vi "Screen Caps VI.vi"() -> ()   [LabVIEW 2015]
uses:
  Circle cluster.ctl
  colors.ctl
  Circle/Circle.lvclass
  Shape/Shape.lvclass/Shape.ctl
  Circle Library.lvlib
  Shape/Shape.lvclass
panel:
  out "area":dbl
  out "area":dbl
  in  "error in (no error)":errorcluster
  out "output cluster":T1
  in  "Radius":dbl
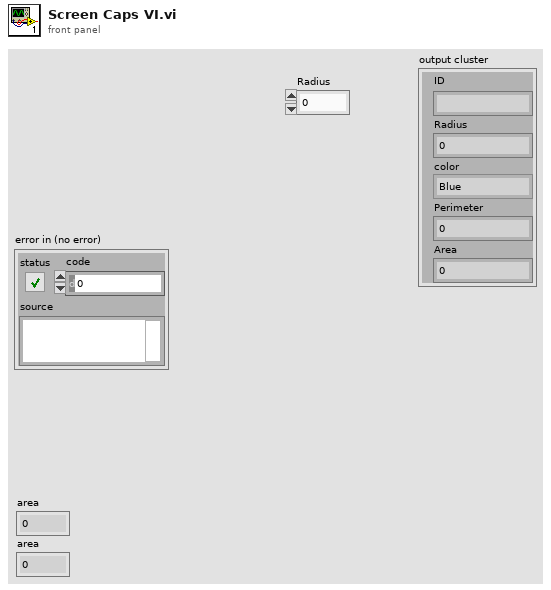
[diagram p1: front panel]
types:
  T1 = typedef "Circle Library.lvlib/Circle cluster.ctl" = cluster{"ID":string, "Radius":dbl, "color":T2, "Perimeter":dbl, "Area":dbl}
  T2 = typedef "colors.ctl" = enum16{"Blue", "Red", "Green", "Yellow"}
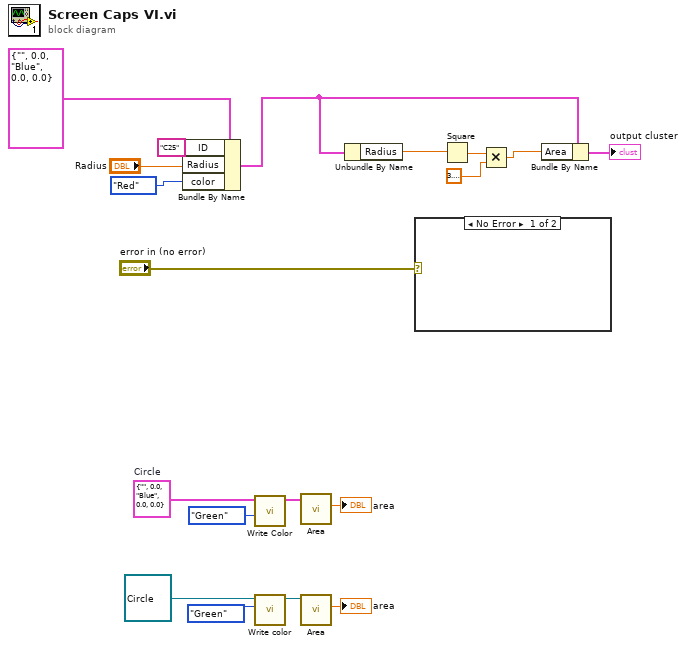
[diagram p0: block diagram]
diagram:
  w6 = T1 {"ID"="", "Radius"=0.0, "color"=enum."Blue", "Perimeter"=0.0, "Area"=0.0}  # Circle
  n1 = Bundle By Name(cluster=T1 {"ID"="", "Radius"=0.0, "color"=enum."Blue", "Perimeter"=0.0, "Area"=0.0} ("Circle"), "ID"="C25", "Radius"="Radius", "color"=colors."Red") -> (w13:T1)
  n2 = call "Write Color.vi"("color"=colors."Green", "Circle"=w6) -> ("Circle 2"=w5:T1)  [unwired: 9 in]
  n3 = call "Write color.vi"("color"=colors."Green", "Shape in"=refnum<class "Circle.lvclass"> refnum ("Circle.lvclass")) -> ("Shape out"=w2:refnum<class "Circle.lvclass">)  [unwired: 8 in, 1 out]
  n4 = call "Area.vi"("Circle in"=w5) -> ("Area"=→"area":dbl)  [unwired: 9 in, 1 out]
  n5 = call-dynamic "Area.vi"("Circle in"=w2) -> ("area"=→"area":dbl)  [unwired: 8 in, 2 out]
  n6 = Unbundle By Name(w13) -> ("Radius"=w18:dbl)
  n7 = case shown="No Error" "error in (no error)" {
    frame No Error {
    }
    frame Error {
    }
  }
  n8 = Square(x=w18) -> (x^2=w17:dbl)
  n9 = Multiply(x=w17, y=3.141592653589793) -> (x*y=w12:dbl)
  n10 = Bundle By Name(cluster=w13, "Area"=w12) -> (→"output cluster":T1)
